vi "SetSyncOption.vi"(1 "SyncOption":T1, 3 "SyncTime(s)":i32, 5 "error in (no error)":errorcluster) -> (19 "error out":errorcluster)   [LabVIEW 2012, in "UmlEditor.lvclass"]
uses:
  <resource>/Framework/Providers/Open_GDS/UML/UmlEditor_class/UmlEditor.lvclass
  <resource>/Framework/Providers/Open_GDS/UML/UMLEditor/UMLEditor_SyncOptions.ctl
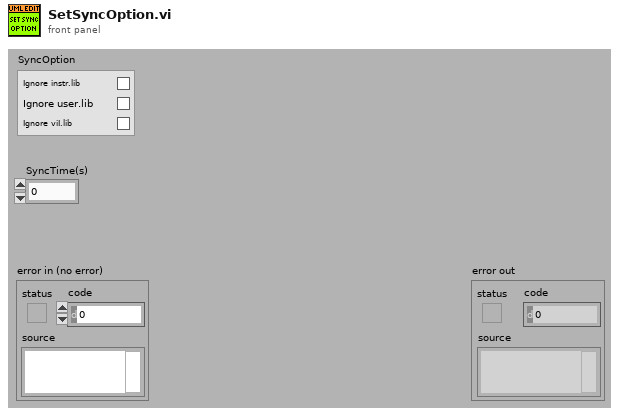
[diagram p1: front panel]
types:
  T1 = typedef "UMLEditor_SyncOptions.ctl" = cluster{"IgnoreInstrLib":bool, "IgnoreUserLib":bool, "IgnoreViLib":bool}
  T2 = typedef "UmlEditor.lvclass/ObjectAttributes.ctl" = cluster{"ListeningQueueIn":refnum<queue>, "Event":refnum<user-event>, "UseProjectFolderAsBasePath":bool, "TypeSyncOption":bool, "Attr":string[], "ToolTip":cluster{"ToolTipOpen":bool, "LastToolTip":i32}, "ClassesToIgnore":string[], "UndoSize":i32, "OpenLastSavedFileWhenStarting":bool, "SyncOption":T1, "SyncTime(s)":i32, "Params":cluster{"IniParams":T3, "Value":string}[]}
  T3 = typedef "UmlEditor.lvclass/IniParamsType.ctl" = enum16{"I have problem with UML stability on my computer"}
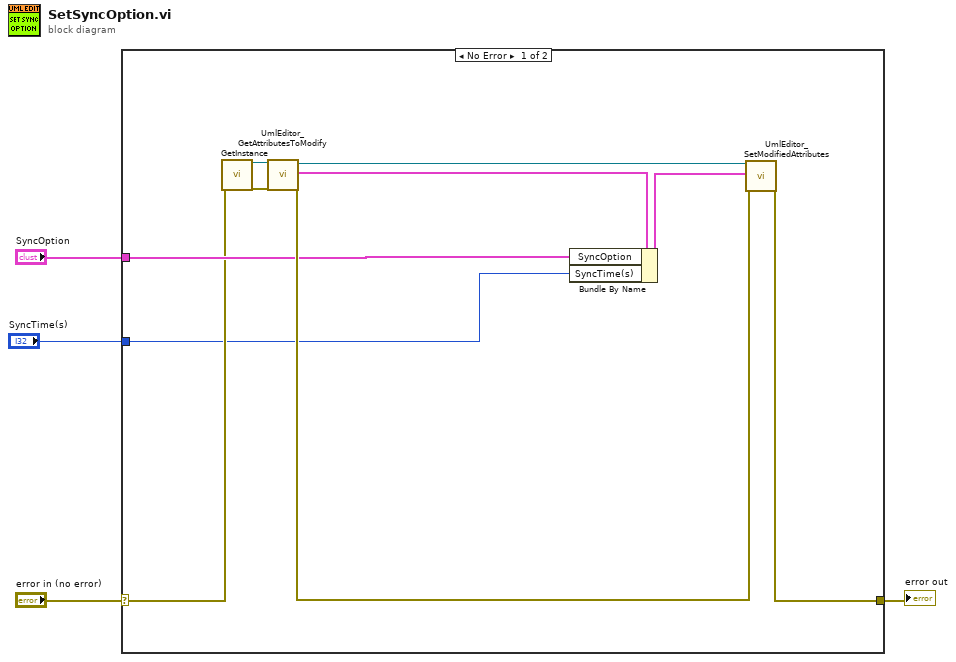
[diagram p0: block diagram]
diagram:
  n1 = case shown="No Error" "error in (no error)" {
    selector: "error in (no error)" -> [w6 w15]
    tunnel: [w11 w15] -> w3
    tunnel: "SyncOption" -> [w9 _]
    tunnel: "SyncTime(s)" -> [w5 _]
    frame No Error {
      n2 = call <resource>:"GetInstance.vi"("error in (no error)"=w6) -> ("reference out"=w8:refnum<class "UmlEditor.lvclass">, "error out"=w7:errorcluster)  [unwired: 17 out]
      n3 = call <resource>:"UmlEditor_GetAttributesToModify.vi"("reference in"=w8, "error in (no error)"=w7) -> ("reference out"=w12:refnum<class "UmlEditor.lvclass">, "Attributes"=w14:T2, "error out"=w10:errorcluster)  [unwired: 14 in, 1 out]
      n4 = Bundle By Name(cluster=w14, "SyncOption"=w9, "SyncTime(s)"=w5) -> (w13:T2)
      n5 = call <resource>:"UmlEditor_SetModifiedAttributes.vi"("reference in"=w12, "Attributes"=w13, "error in (no error)"=w10) -> ("error out"=w11:errorcluster)  [unwired: 15 in, 1 out]
    }
    frame Error {
    }
  }
  "error out" <- w3
